vi "RT File IO.vi"() -> ()   [LabVIEW 2026]
panel:
  out "path 2":path
  out "path":path
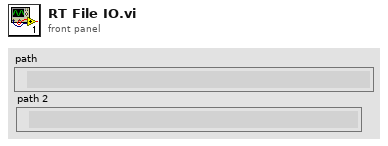
[diagram p1: front panel]
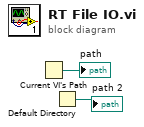
[diagram p0: block diagram]
diagram:
  n1 = Current VI's Path() -> (path=→"path":path)
  n2 = Default Directory() -> (→"path 2":path)
